vi "BRig_Host__Loop_Consumer_RunState__updatePlot__plotData_get.vi"(5 "input_idx":i32[](array[numeric]), 7 "input_dataPlot":u16[][](array[numeric])) -> (2 "output_plotData":cluster{u16[], u16[]}[](array[cluster]))   [LabVIEW 2014]
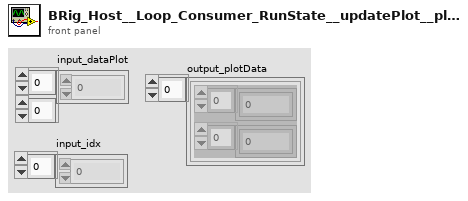
[diagram p1: front panel]
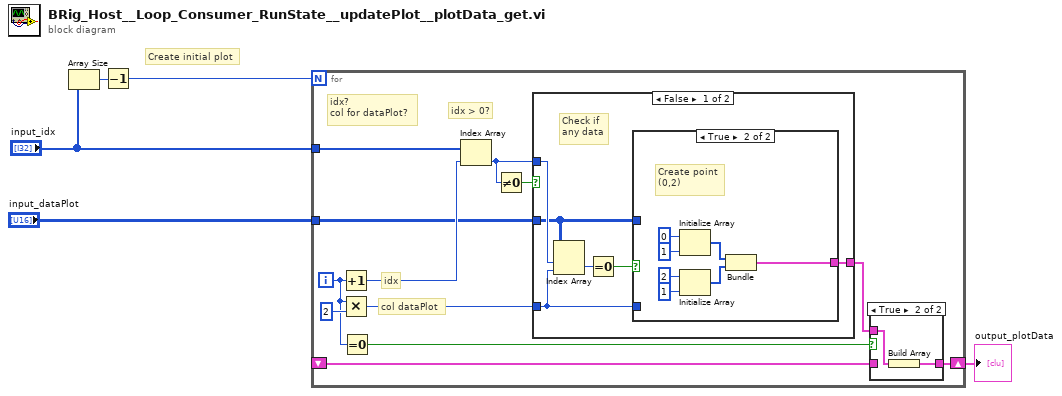
[diagram p0: block diagram]
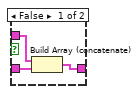
[diagram p2: hidden frame]
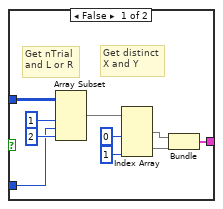
[diagram p3: hidden frame]
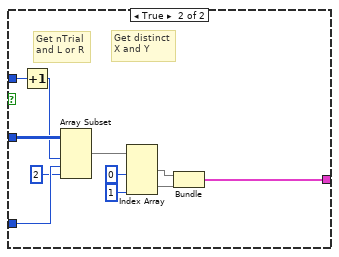
[diagram p4: hidden frame]
diagram:
  # "Create initial plot"
  n1 = Array Size(array="input_idx") -> (size(s)=w5:i32)
  n2 = Decrement(x=w5) -> (x-1=w1:i32)
  n3 = for {
    N: w1 -> [_]
    tunnel: "input_idx" -> [w17]
    tunnel: "input_dataPlot" -> [w11]
    shift-right: [w7] -> w2
    shift-left: _ -> [w6]
    i -> [w14]
    # "col dataPlot"
    # "idx"
    # "idx > 0?"
    # "idx?\ncol for dataPlot?"
    n4 = Increment(x=w14) -> (x+1=w16:i32)
    n5 = Multiply(x=w14, y=2) -> (x*y=w10:i32)
    n6 = Equal To 0?(x=w14) -> (x = 0?=w9:bool)
    n7 = Index Array(array=w17, index=w16) -> (element=w12:i32)
    n8 = Not Equal To 0?(x=w12) -> (x != 0?=w13:bool)
    n9 = case shown="False" w13 {
      tunnel: w12 -> [w28 w55]
      tunnel: w11 -> [w25 w56]
      tunnel: w10 -> [w24 w53]
      tunnel: [w23 w46] -> w8
      frame False {
        # "Check if\nany data"
        n10 = Index Array(array=w25, index (row)=w28, index (col)=w24) -> (element=w27:u16)
        n11 = Equal To 0?(x=w27) -> (x = 0?=w26:bool)
        n12 = case shown="True" w26 {
          tunnel: w25 -> [w32 _]
          tunnel: w24 -> [w30 _]
          tunnel: [w29 w39] -> w23
          frame False {
            # "Get distinct\nX and Y"
            # "Get nTrial\nand L or R"
            n13 = Array Subset(array=w32, length (row)=1 ("length"), index (col)=w30, length (col)=2 ("length")) -> (w33:u16[][])  [unwired: 1 in]
            n14 = Index Array(array=w33, index (col) #1=0 ("disabled index (col)"), index (col) #2=1 ("index (col)")) -> (element #1=w35:u16[], element #2=w34:u16[])  [unwired: 2 in]
            n15 = Bundle(w35, w34) -> (w29:cluster{u16[], u16[]})  [unwired: 1 in]
          }
          frame True {
            # "Create point\n(0,2)"
            n16 = Initialize Array(u16 0 ("element"), 1 ("dimension size")) -> (w41:u16[])
            n17 = Initialize Array(u16 2 ("element"), 1 ("dimension size")) -> (w40:u16[])
            n18 = Bundle(w41, w40) -> (w39:cluster{u16[], u16[]})  [unwired: 1 in]
          }
        }
      }
      frame True {
        # "Get distinct\nX and Y"
        # "Get nTrial\nand L or R"
        n19 = Increment(x=w55) -> (x+1=w54:i32)
        n20 = Array Subset(array=w56, length (row)=w54, index (col)=w53, length (col)=2 ("length")) -> (w47:u16[][])  [unwired: 1 in]
        n21 = Index Array(array=w47, index (col) #1=0 ("disabled index (col)"), index (col) #2=1 ("index (col)")) -> (element #1=w49:u16[], element #2=w48:u16[])  [unwired: 2 in]
        n22 = Bundle(w49, w48) -> (w46:cluster{u16[], u16[]})  [unwired: 1 in]
      }
    }
    n23 = case shown="True" w9 {
      tunnel: w8 -> [w19 w22]
      tunnel: [w20 w21] -> w7
      tunnel: w6 -> [w18 _]
      frame False {
        n24 = Build Array (concatenate)(w19, w18) -> (w20:cluster{u16[], u16[]}[])
      }
      frame True {
        n25 = Build Array(w22) -> (w21:cluster{u16[], u16[]}[])
      }
    }
  }
  "output_plotData" <- w2
